vi "Check Last Step.vi"(8 "Error In":errorcluster, 11 "reference in":refnum<class "Recipe.lvclass">) -> (0 "Error Out":errorcluster, 2 "Is Last Step":bool, 3 "reference out":refnum<class "Recipe.lvclass">)   [LabVIEW 2021, in "Recipe.lvclass"]
uses:
  Recipe.lvclass
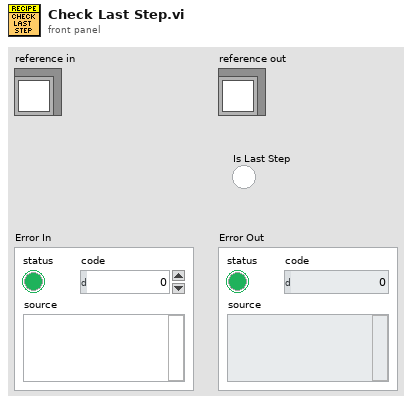
[diagram p1: front panel]
types:
  T1 = typedef "Recipe.lvclass/ObjectAttributes.ctl" = cluster{"Steps":refnum<class "Recipe Step.lvclass">[], "Current Info":cluster{"Current Index":u64}}
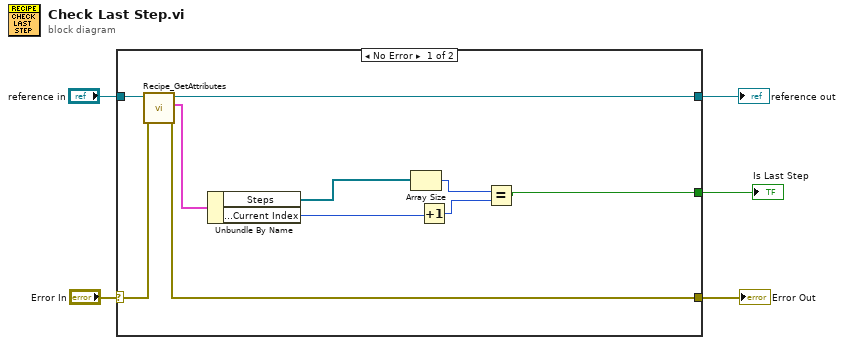
[diagram p0: block diagram]
diagram:
  n1 = case shown="No Error" "Error In" {
    selector: "Error In" -> [w15 w17]
    tunnel: [w13 w17] -> w4
    tunnel: [w11 w16] -> w2
    tunnel: "reference in" -> [w12 w16]
    tunnel: [w6 _] -> w1
    frame No Error {
      n2 = call "Recipe_GetAttributes.vi"("Error In"=w15, "reference in"=w12) -> ("Error Out"=w13:errorcluster, "Data"=w14:T1, "reference out"=w11:refnum<class "Recipe.lvclass">)  [unwired: 6 in, 1 out]
      n3 = Unbundle By Name(w14) -> ("Steps"=w10:refnum<class "Recipe Step.lvclass">[], "Current Info.Current Index"=w9:u64)
      n4 = Array Size(array=w10) -> (size(s)=w7:i32)
      n5 = Increment(x=w9) -> (x+1=w8:u64)
      n6 = Equal?(x=w7, y=w8) -> (x = y?=w6:bool)
    }
    frame Error {
    }
  }
  "Error Out" <- w4
  "reference out" <- w2
  "Is Last Step" <- w1
